vi "ecg_ncs_v1a.vi"() -> ()   [LabVIEW 2016]
uses:
  <instrlib>/niUSRP/niUSRP Timestamp.ctl
  C:/Program Files/National Instruments/LabVIEW 2016/examples/Instrument IO/Serial/support/Serial - Settings.ctl
  <vilib>/Analysis/coordinate.llb/Wrap Angle (array).vi
  <instrlib>/niUSRP/niUSRP Configure Time Start Trigger.vi
  <vilib>/Instr/_visa.llb/VISA Configure Serial Port (Instr).vi
  <instrlib>/niUSRP/niUSRP Fetch Rx Data (2D CDB).vi
  <vilib>/Analysis/3filter.llb/Butterworth Filter (DBL).vi
  <instrlib>/niUSRP/niUSRP Write Tx Data (2D CDB).vi
  <vilib>/measure/NI_MABase.lvlib
  <vilib>/Analysis/NI_AALBase.lvlib
  <vilib>/Analysis/NI_AALPro.lvlib
  <vilib>/Analysis/NI_AAL_Angle.lvlib
panel:
  out "Iteration visa":i32=2074
  in  "?":enum32{"ECG", "Heart Rate"}(tab)
  out "BMD101 Reading":i16[](graph)=[10]
  out "Heart Rate":u8[](graph)=[100]
  in  "Read Count":u32=24
  out "return count":u32=8
  out "Poor Sensor Quality: \nSensor off":bool=TRUE
  out "Poor Sensor Quality: \nSensor on":bool
  out "Heart Rate 2":u16[](array[numeric])=[100]
  out "Stop Loop":bool=TRUE
  in  "Read":bool=TRUE
  in  "Stop":bool
  in  "Serial Settings":T1={"baud rate"=57600, "data bits"=8, "parity"=enum."None", "stop bits"=10, "flow control"=0} {"flow control" items=["None"=0, "XON/XOFF"=1, "RTS/CTS"=2, "DTR/DSR"=4]; "stop bits" items=["1.0"=10, "1.5"=15, "2.0"=20]; "data bits" min=5 max=8 step=1; "baud rate" items=["75"=75, "110"=110, "134"=134, "150"=150, "300"=300, "600"=600, "1200"=1200, "1800"=1800, "2400"=2400, "4800"=4800, "7200"=7200, "9600"=9600, "14400"=14400, "19200"=19200, "28800"=28800, "38400"=38400, "56000"=56000, "57600"=57600, "115200"=115200, "128000"=128000, "230400"=230400]}
  in  "VISA resource name":refnum<visa-resource-name>="bmd101"
  in  "File Name":string="Test"
  in  "order1":i32=5
  in  "Path":path=path "D:/Research/SummerFall17Spring18/CnC/NCS/EcgNcsCorrelation"
  in  "Low-Pass Freq":dbl=200.0 format="%#_13g"
  in  "Sampling Rate":i32=500
  out "Gain":dbl=-15.0
  out "Bandwidth":dbl=56000000.0
  out "Coerced Carrier Frequency":dbl=2000000000.0 format="%#.17g"
  out "Coerced Tx IQ rate":dbl=1000000.0
  out "Coerced Rx IQ rate":dbl=1000000.0
  out "error IO":errorcluster={"status"=FALSE, "code"=-1074118647, "source"=""}
  in  "Rx Number of Samples":i32=20000
  in  "Tab Control 2":enum32{"NI-294x/295x", "NI-2900/2901"}(tab)=enum."NI-2900/2901"
  in  "channel 0 carrier\n frequency [Hz]":dbl=2000000000.0 format="%#_6p"
  in  "Rx carrier frequency [Hz]":dbl=2000000000.0 format="%#_6p"
  in  "Tx carrier frequency [Hz]":dbl=1000000000.0 format="%#_6p"
  in  "Start Trigger Time":T2={"whole seconds"=1, "fractional seconds"=0.0}
  out "Tx Active Antenna":string="TX1"
  in  "Tab Control":T3(tab)
  out "NCS tag Amp":dbl[](graph)=[0.013332788438327721, 0.0131552898712497, 0.012994905519721597, 0.012986271887777701, 0.013075284595455733, 0.013191204808537919, 0.013351894528100879, 0.01345386740636616, 0.013382234051438232, 0.013180163786137358]
  out "NCS tag Phase":dbl[](graph)=[114.08993023907641, 111.82225141412982, 110.02998222947944, 109.41153055749608, 110.12587965469353, 112.16042160734105, 113.81215100166591, 114.51260226782536, 113.6206368361215, 111.46787264294511]
  out "IQ":dbl[][](graph)
  out "Tag Amp":dbl[](graph)
  out "Tag Phase":dbl[](graph)
  out "Tx Waveform Graph":waveform(dbl)[](graph)=[{"t0"=timestamp(0 s since 1904-01-01), "dt"=1e-06, "Y"=array[2000 elements]}, {"t0"=timestamp(0 s since 1904-01-01), "dt"=1e-06, "Y"=array[2000 elements]}]
  in  "Channel 0\nTone Amplitude":dbl=0.707 step=0.05 format="%#.6g"
  in  "Channel 0 \nTone Frequency":dbl=5000.0 format="%#_6p"
  in  "Waveform Size":dbl=2000.0
  in  "Rx Active Antenna":string="RX2"
  in  "Device Name":refnum<k15>="MyB200"
  in  "Tx Gain":dbl=28.0 format="%#_6f"
  in  "Tx IQ Rate":dbl=1000000.0 format="%#_6p"
  in  "Rx Gain":dbl=32.0 format="%#_6f"
  in  "Rx IQ Rate":dbl=1000000.0 format="%#_6p"
  # "Rx Settings"
  # "Tx Settings"
  # "Note that on the NI-2900 and NI-2901, both Rx channels share an LO and both Tx channels share an LO. However, on the NI-294x/295x devices, Rx and Tx of channel 0 share an LO and Rx and Tx of channel 1 share an LO."
  # "This Tx graph should always have end and start tied up since this is being sent in a loop continuously. Otherwise phase jumps will be noticed."
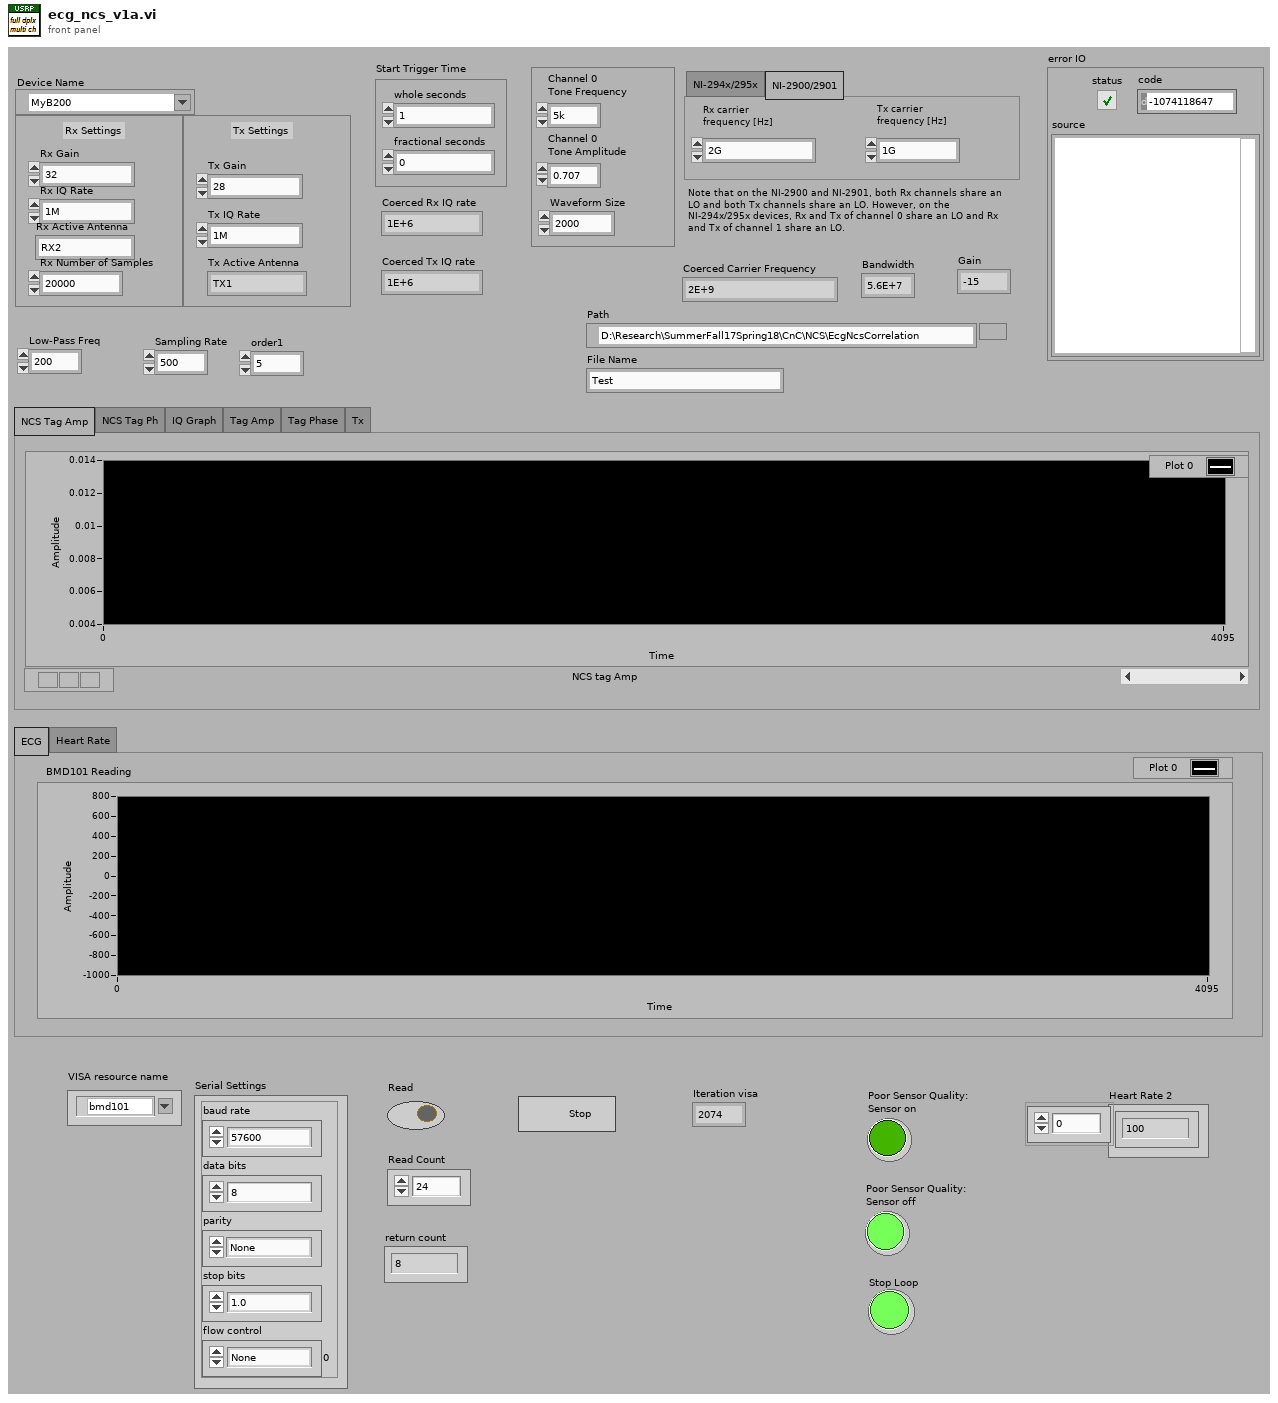
[diagram p1: front panel]
types:
  T1 = typedef "Serial - Settings.ctl" = cluster{"baud rate":u32, "data bits":u16, "parity":enum16{"None", "Odd", "Even", "Mark", "Space"}, "stop bits":u16, "flow control":u16}
  T2 = typedef "niUSRP Timestamp.ctl" = cluster{"whole seconds":u64, "fractional seconds":dbl}
  T3 = enum32{"NCS Tag Amp", "NCS Tag Ph", "IQ Graph", "Tag Amp", "Tag Phase", "Tx"}
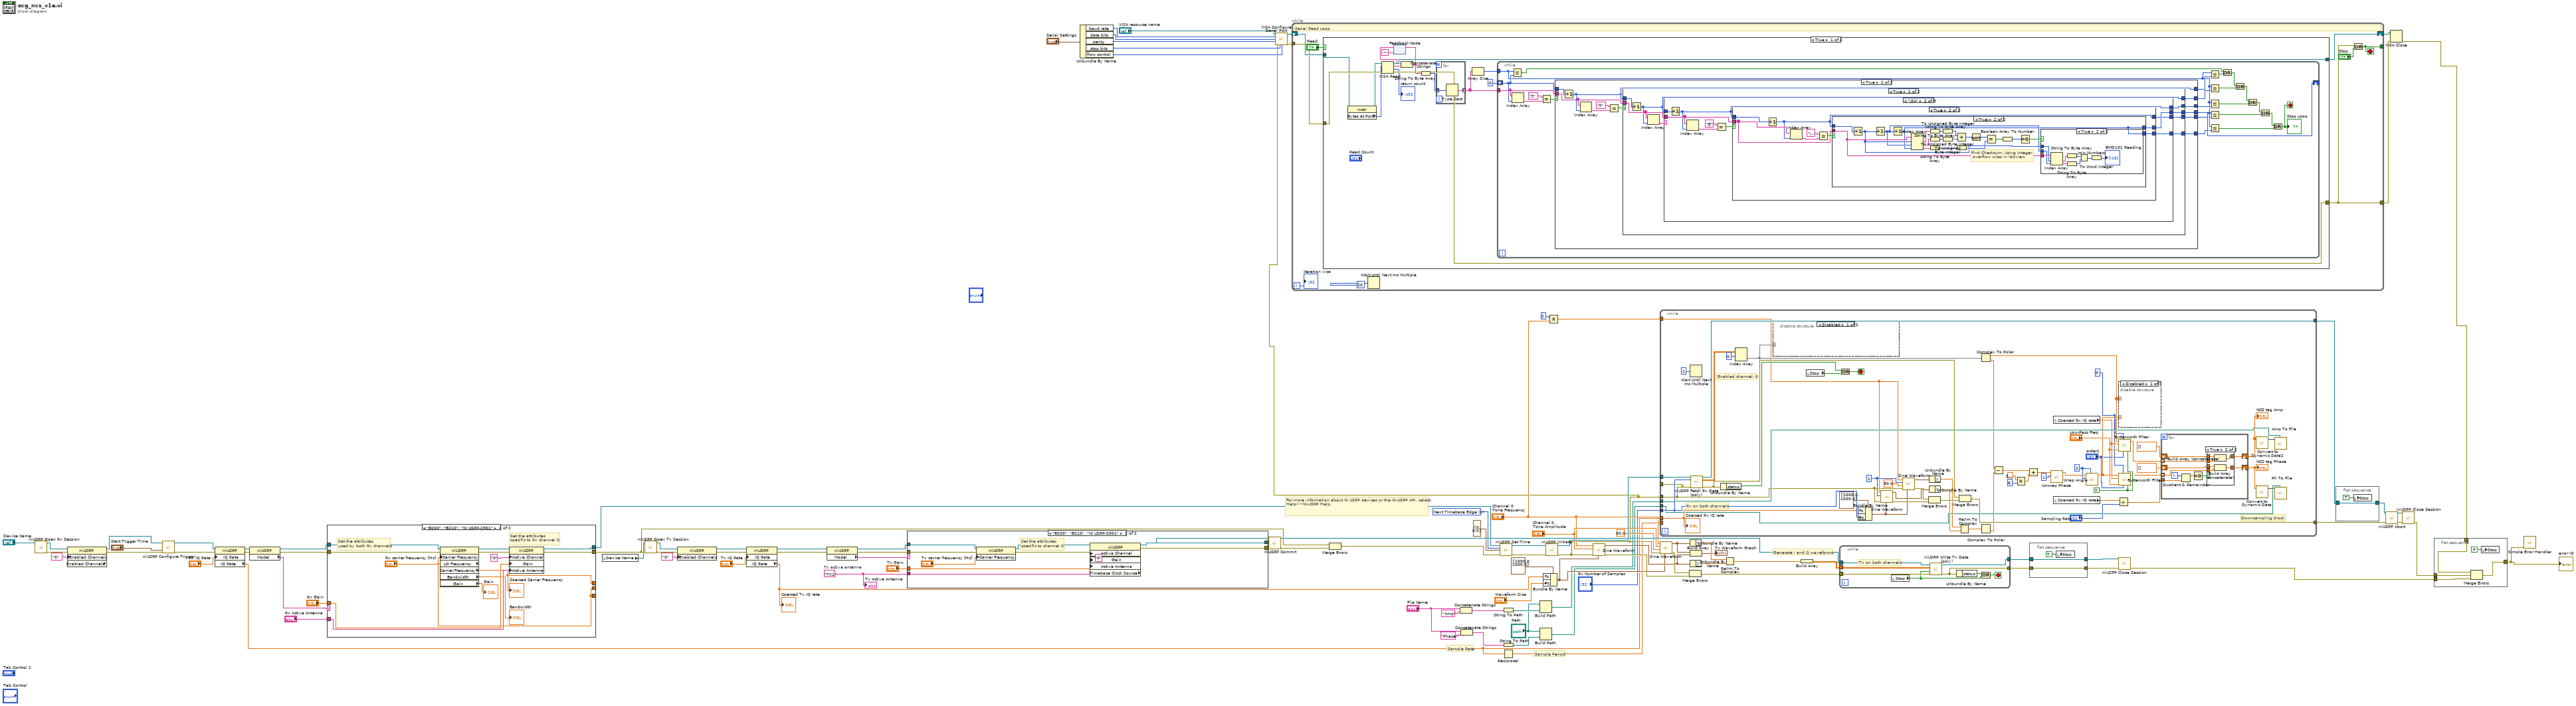
[diagram p0: block diagram]
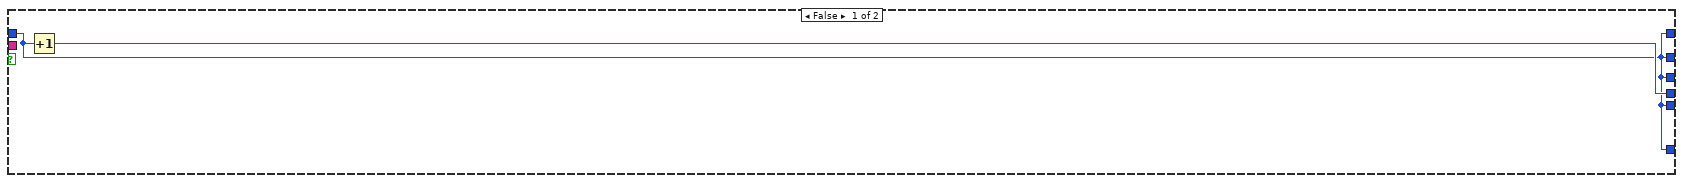
[diagram p2: hidden frame]
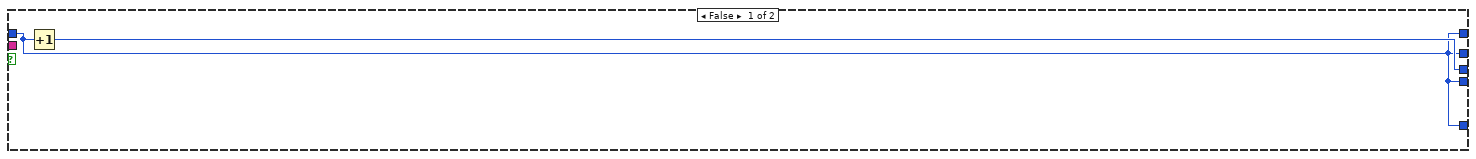
[diagram p3: hidden frame]
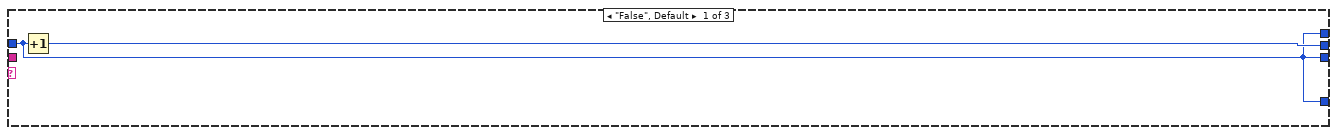
[diagram p4: hidden frame]
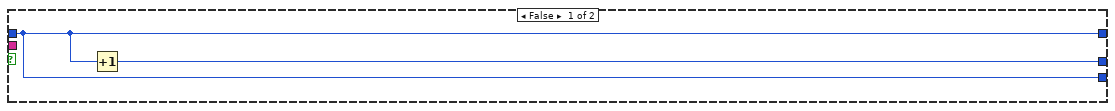
[diagram p5: hidden frame]
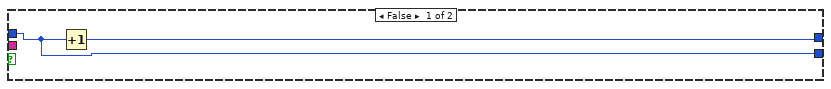
[diagram p6: hidden frame]
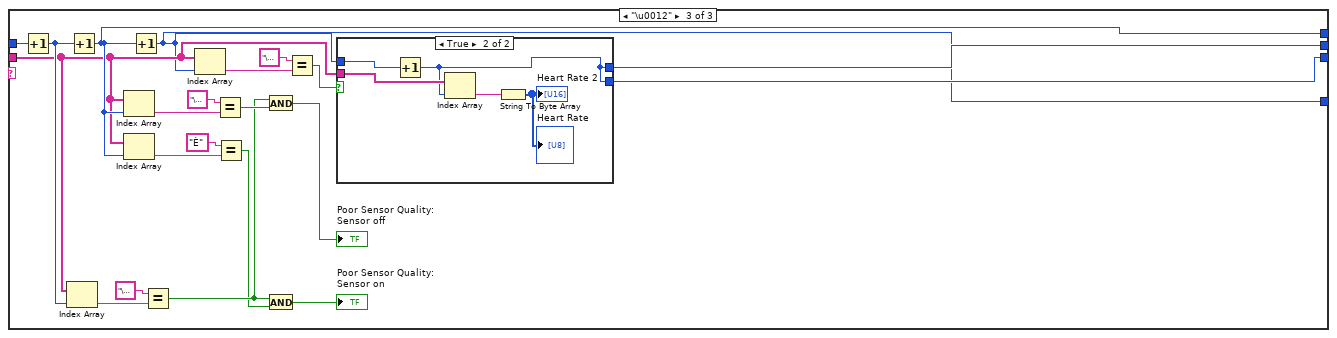
[diagram p8: hidden frame]
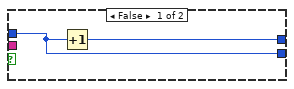
[diagram p9: hidden frame]
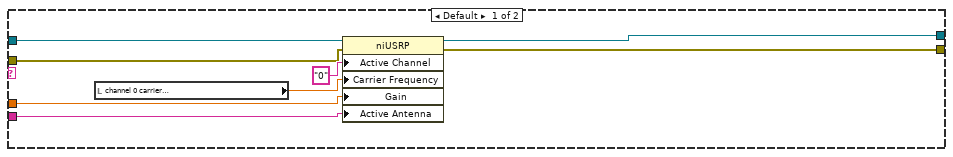
[diagram p11: hidden frame]
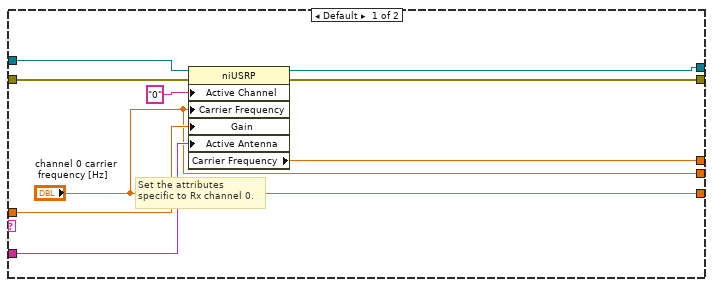
[diagram p12: hidden frame]
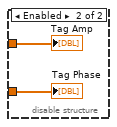
[diagram p13: hidden frame]
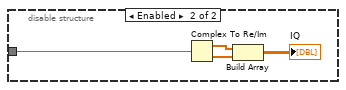
[diagram p14: hidden frame]
diagram:
  w73 = 1 items=["Now", "Next Timebase Edge"] ("apply timestamp")
  w42 = "TX1"  # Tx active antenna
  # "Sample Rate"
  # "Sample Period"
  # "For more information about NI USRP devices or the NI-USRP API, select Help>>NI-USRP Help."
  # "Generate I and Q waveforms."
  n1 = call <instrlib>:"niUSRP Open Rx Session.vi"("device names"="Device Name") -> ("session handle out"=w72:refnum<k15>, "error out"=w71:errorcluster)  [unwired: 13 in]
  n2 = property class="niUSRP" props=["Enabled Channels", "Enabled Channels"](reference=w72, error in=w71, "Enabled Channels"="0" ("Configuration:Enabled Channels")) -> (reference out=w70:refnum<k15>, error out=w69:errorcluster)  [unwired: 1 out]
  n3 = call-poly <instrlib>:"niUSRP Configure Trigger.vi"("session handle"=w70, "start trigger time"="Start Trigger Time", "error in (no error)"=w69) -> ("session handle out"=w66:refnum<k15>, "error out"=w65:errorcluster)  [unwired: 11 in]
  n4 = property class="niUSRP"(reference=w66, error in=w65, "IQ Rate"="Rx IQ Rate") -> (reference out=w62:refnum<k15>, error out=w63:errorcluster, "IQ Rate"=w29:dbl)
  n5 = property class="niUSRP"(reference=w62, error in=w63) -> (reference out=w57:refnum<k15>, error out=w58:errorcluster, "Model"=w59:string)
  n6 = case shown="\"B200\", \"B210\", \"NI USRP-2901\"" w59 {
    tunnel: w58 -> [w108 w118]
    tunnel: w57 -> [w107 w119]
    tunnel: [w104 w115] -> w61
    tunnel: [w103 w114] -> w60
    tunnel: "Rx Gain" -> [w106 w121]
    tunnel: "Rx Active Antenna" -> [w105 w120]
    tunnel: [w101 w110] -> _
    tunnel: ["channel 0 carrier\n frequency [Hz]" "Rx carrier frequency [Hz]"] -> _
    tunnel: ["channel 0 carrier\n frequency [Hz]" "Rx carrier frequency [Hz]"] -> _
    frame Default {
      # "Set the attributes \nspecific to Rx channel 0."
      n7 = property class="niUSRP"(reference=w107, error in=w108, "Active Channel"="0", "Carrier Frequency"="channel 0 carrier\n frequency [Hz]", "Gain"=w106, "Active Antenna"=w105) -> (reference out=w104:refnum<k15>, error out=w103:errorcluster, "Carrier Frequency"=w101:dbl)
    }
    frame "B200", "B210", "NI USRP-2901" {
      # "Set the attributes \nused by both Rx channels"
      # "Set the attributes \nspecific to Rx channel 0."
      n8 = property class="niUSRP" props=["Carrier Frequency", "LO Frequency", "Carrier Frequency", "Bandwidth", "Gain"](reference=w119, error in=w118, "Carrier Frequency"="Rx carrier frequency [Hz]") -> (reference out=w117:refnum<k15>, error out=w116:errorcluster, "Carrier Frequency"=w110:dbl, "Bandwidth"=→"Bandwidth":dbl, "Gain"=→"Gain":dbl)  [unwired: 1 out]
      "Coerced Carrier Frequency" <- w110
      n9 = property class="niUSRP"(reference=w117, error in=w116, "Active Channel"="0", "Gain"=w121, "Active Antenna"=w120) -> (reference out=w115:refnum<k15>, error out=w114:errorcluster)
    }
  }
  n10 = local read "Device Name"() -> (w94:refnum<k15>)
  n11 = call <instrlib>:"niUSRP Open Tx Session.vi"("device names"=w94, "error in (no error)"=w60) -> ("session handle out"=w68:refnum<k15>, "error out"=w67:errorcluster)  [unwired: 12 in]
  n12 = property class="niUSRP"(reference=w68, error in=w67, "Enabled Channels"="0" ("Configuration:Enabled Channels")) -> (reference out=w54:refnum<k15>, error out=w53:errorcluster)
  n13 = property class="niUSRP"(reference=w54, error in=w53, "IQ Rate"="Tx IQ Rate") -> (reference out=w48:refnum<k15>, error out=w49:errorcluster, "IQ Rate"=w46:dbl)
  "Coerced Tx IQ rate" <- w46
  n14 = property class="niUSRP"(reference=w48, error in=w49) -> (reference out=w50:refnum<k15>, error out=w51:errorcluster, "Model"=w47:string)
  n15 = case shown="\"B200\", \"B210\", \"NI USRP-2901\"" w47 {
    tunnel: "Tx Gain" -> [w130 w140]
    tunnel: w42 -> [w128 w138]
    tunnel: [w124 w132] -> w44
    tunnel: [w123 w131] -> w45
    tunnel: w51 -> [w127 w134]
    tunnel: w50 -> [w126 w137]
    frame Default {
      n16 = local read "channel 0 carrier\n frequency [Hz]"() -> (w125:dbl)
      n17 = property class="niUSRP"(reference=w126, error in=w127, "Active Channel"="0", "Carrier Frequency"=w125, "Gain"=w130, "Active Antenna"=w128) -> (reference out=w124:refnum<k15>, error out=w123:errorcluster)
    }
    frame "B200", "B210", "NI USRP-2901" {
      # "Set the attributes \nspecific to channel 0."
      n18 = property class="niUSRP"(reference=w137, error in=w134, "Carrier Frequency"="Tx carrier frequency [Hz]") -> (reference out=w136:refnum<k15>, error out=w135:errorcluster)
      n19 = property class="niUSRP" props=["Active Channel", "Gain", "Active Antenna", "Timebase Clock Source"](reference=w136, error in=w135, "Active Channel"="0", "Gain"=w140, "Active Antenna"=w138) -> (reference out=w132:refnum<k15>, error out=w131:errorcluster)  [unwired: 1 out]
    }
  }
  n20 = Unbundle By Name("Serial Settings") -> ("baud rate"=w13:u32, "data bits"=w12:u16, "parity"=w11:enum16{"None", "Odd", "Even", "Mark", "Space"}, "stop bits"=w10:u16, "flow control"=w9:u16)
  n21 = call <instrlib>:"niUSRP Commit.vi"("session handle"=w44, "error in (no error)"=w45) -> ("session handle out"=w96:refnum<k15>, "error out"=w97:errorcluster)  [unwired: 12 in]
  n22 = Merge Errors(w60, w97) -> (w75:errorcluster)
  n23 = Concatenate Strings("File Name", "Amp") -> (w22:string)
  n24 = Concatenate Strings("File Name", "Phase") -> (w18:string)
  n25 = call <instrlib>:"niUSRP Set Time.vi"("session handle"=w61, "apply timestamp"=w73, "timestamp"=T2 {"whole seconds"=0, "fractional seconds"=0.0}, "error in (no error)"=w75) -> ("session handle out"=w77:refnum<k15>, "error out"=w76:errorcluster)  [unwired: 10 in]
  n26 = String To Path(string=w22) -> (path=w21:path)
  n27 = String To Path(string=w18) -> (path=w17:path)
  n28 = Reciprocal(x=w29) -> (1/x=w80:dbl)
  n29 = Build Path(base path="Path", name or relative path=w21) -> (appended path=w24:path)
  n30 = Build Path(base path="Path", name or relative path=w17) -> (appended path=w15:path)
  n31 = Bundle By Name(cluster=cluster{"Fs":dbl, "#s":dbl} {"Fs"=1000.0, "#s"=1000.0} ("sampling info"), "Fs"=w46, "#s"="Waveform Size") -> (w79:cluster{"Fs":dbl, "#s":dbl})
  n32 = call <instrlib>:"niUSRP Initiate.vi"("session handle"=w77, "error in (no error)"=w76) -> ("session handle out"=w100:refnum<k15>, "error out"=w3:errorcluster)  [unwired: 12 in]
  n33 = call-poly "VISA Configure Serial Port"("VISA resource name"="VISA resource name", "baud rate (9600)"=w13, "data bits (8)"=w12, "parity (0:none)"=w11, "error in (no error)"=w3, "stop bits (10: 1 bit)"=w10, "flow control (0:none)"=w9) -> ("VISA resource name out"=w6:refnum<visa-resource-name>, "error out"=w5:errorcluster)  [unwired: 3 in, 4 out]
  n34 = while {
    shift-right: [w149] -> w7
    shift-left: w6 -> [w147]
    tunnel: w5 -> [w143]
    tunnel: [w146] -> _
    tunnel: [w142] -> w1
    i -> [w141]
    stop <- w146 stop-if-true
    # "Serial Read Loop"
    n35 = case shown="True" "Read" {
      tunnel: [w164 w293] -> w149
      tunnel: w147 -> [w152 w293]
      tunnel: [w153 w292] -> w142
      tunnel: w143 -> [w154 w292]
      frame True {
        n36 = property class="Instr"(reference=w152) -> (reference out=w151:refnum<visa-resource-name>, "Bytes at Port"=w150:u32)  [unwired: 1 in, 1 out]
        n37 = VISA Read(VISA resource name=w151, byte count=w150, error in (no error)=w154) -> (VISA resource name out=w164:refnum<visa-resource-name>, read buffer=w163:string, return count=→"return count":u32, error out=w153:errorcluster)
        n38 = feedback #1("") -> (w162:string)
        n39 = Concatenate Strings(w162, w163) -> (w159:string)
        n40 = feedback-in #1(w159) -> ()
        n41 = String To Byte Array(string=w159) -> (unsigned byte array=w160:u8[])
        n42 = for {
          tunnel: w160 -> [w291] mode=indexing
          tunnel: [w290] -> w157 mode=indexing
          n43 = Type Cast(x=w291) -> (*(type *) &x=w290:string)  [unwired: 1 in]
        }
        n44 = Array Size(array=w157) -> (size(s)=w155:i32)
        n45 = while {
          tunnel: w157 -> [w183]
          shift-right: [w187] -> _
          shift-left: 0 -> [w182]
          tunnel: w155 -> [w168]
          stop <- w165 stop-if-true
          n46 = Less Or Equal?(x=w168, y=w182) -> (x <= y?=w180:bool)
          n47 = Index Array(array=w183, index=w182) -> (element=w186:string)
          n48 = Equal?(x="ª", y=w186) -> (x = y?=w184:bool)
          n49 = case shown="True" w184 {
            tunnel: w182 -> [w188 w198]
            tunnel: [w189 w196] -> w187
            tunnel: w183 -> [_ w190]
            tunnel: [w188 w195] -> w181
            tunnel: [w188 w194] -> w178
            tunnel: [w188 w193] -> w175
            tunnel: [w188 w192] -> w172
            tunnel: [w188 w191] -> w169
            frame False {
              n50 = Increment(x=w188) -> (x+1=w189:i32)
            }
            frame True {
              n51 = Increment(x=w198) -> (x+1=w195:i32)
              n52 = Index Array(array=w190, index=w195) -> (element=w200:string)
              n53 = Equal?(x="ª", y=w200) -> (x = y?=w197:bool)
              n54 = case shown="True" w197 {
                tunnel: w195 -> [w201 w204]
                tunnel: [w202 w210] -> w196
                tunnel: w190 -> [_ w209]
                tunnel: [w201 w205] -> w194
                tunnel: [w201 w208] -> w193
                tunnel: [w201 w207] -> w192
                tunnel: [w201 w206] -> w191
                frame False {
                  n55 = Increment(x=w201) -> (x+1=w202:i32)
                }
                frame True {
                  n56 = Increment(x=w204) -> (x+1=w205:i32)
                  n57 = Index Array(array=w209, index=w205) -> (element=w203:string)
                  n58 = case shown="\"\\04\"" w203 {
                    tunnel: w205 -> [w211 w218 w281]
                    tunnel: [w212 w217 w263] -> w210
                    tunnel: w209 -> [_ w216 w265]
                    tunnel: [w211 w215 w267] -> w208
                    tunnel: [w211 w214 w264] -> w207
                    tunnel: [w211 w213 w262] -> w206
                    frame "False", Default {
                      n59 = Increment(x=w211) -> (x+1=w212:i32)
                    }
                    frame "\u0004" {
                      n60 = Increment(x=w218) -> (x+1=w215:i32)
                      n61 = Index Array(array=w216, index=w215) -> (element=w219:string)
                      n62 = Equal?(x="€", y=w219) -> (x = y?=w220:bool)
                      n63 = case shown="True" w220 {
                        tunnel: w215 -> [w222 w228]
                        tunnel: [w223 w227] -> w217
                        tunnel: w216 -> [_ w226]
                        tunnel: [w222 w225] -> w214
                        tunnel: [w222 w224] -> w213
                        frame False {
                          n64 = Increment(x=w222) -> (x+1=w223:i32)
                        }
                        frame True {
                          n65 = Increment(x=w228) -> (x+1=w225:i32)
                          n66 = Index Array(array=w226, index=w225) -> (element=w229:string)
                          n67 = Equal?(x="\u0002", y=w229) -> (x = y?=w230:bool)
                          n68 = case shown="True" w230 {
                            tunnel: w225 -> [w232 w237]
                            tunnel: [w233 w234] -> w227
                            tunnel: w226 -> [_ w238]
                            tunnel: [w232 w234] -> w224
                            frame False {
                              n69 = Increment(x=w232) -> (x+1=w233:i32)
                            }
                            frame True {
                              # "Find Checksum: Using Integer\n overflow rules in labview"
                              n70 = Increment(x=w237) -> (x+1=w236:i32)
                              n71 = Increment(x=w236) -> (x+1=w235:i32)
                              n72 = Increment(x=w235) -> (x+1=w234:i32)
                              n73 = Index Array(array=w238, index #1=w236, index #2=w235, index #3=w234) -> (element #1=w252:string, element #2=w251:string, element #3=w245:string)
                              n74 = String To Byte Array(string=w252) -> (unsigned byte array=w250:u8[])
                              n75 = String To Byte Array(string=w251) -> (unsigned byte array=w249:u8[])
                              n76 = String To Byte Array(string=w245) -> (unsigned byte array=w244:u8[])
                              n77 = To Unsigned Byte Integer(number=w250) -> (unsigned 8bit integer=w248:u8[])
                              n78 = To Unsigned Byte Integer(number=w249) -> (unsigned 8bit integer=w247:u8[])
                              n79 = Add(x=w248, y=w247) -> (x+y=w246:u8[])
                              n80 = To Unsigned Byte Integer(number=w244) -> (unsigned 8bit integer=w242:u8[])
                              n81 = Not(x=w246) -> (.not. x?=w243:u8[])
                              n82 = Equal?(x=w243, y=w242) -> (x = y?=w241:bool[])
                              n83 = Boolean Array To Number(Boolean array=w241) -> (number=w240:u32)
                              n84 = Equal To 0?(x=w240) -> (x = 0?=w239:bool)
                              n85 = case shown="True" w239 {
                                tunnel: w238 -> [_ w261]
                                tunnel: w236 -> [_ w254]
                                tunnel: w235 -> [_ w253]
                                frame False {
                                }
                                frame True {
                                n86 = Index Array(array=w261, index #1=w254, index #2=w253) -> (element #1=w260:string, element #2=w259:string)
                                n87 = String To Byte Array(string=w260) -> (unsigned byte array=w258:u8[])
                                n88 = String To Byte Array(string=w259) -> (unsigned byte array=w257:u8[])
                                n89 = Join Numbers(hi=w258, lo=w257) -> ((hi.lo)=w256:u16[])
                                n90 = To Word Integer(number=w256) -> (16bit integer=→"BMD101 Reading":i16[])
                                }
                              }
                            }
                          }
                        }
                      }
                    }
                    frame "\u0012" {
                      n91 = Increment(x=w281) -> (x+1=w277:i32)
                      n92 = Index Array(array=w265, index=w277) -> (element=w280:string)
                      n93 = Increment(x=w277) -> (x+1=w267:i32)
                      n94 = Index Array(array=w265, index=w267) -> (element=w278:string)
                      n95 = Index Array(array=w265, index=w267) -> (element=w275:string)
                      n96 = Increment(x=w267) -> (x+1=w262:i32)
                      n97 = Equal?(x="\u0002", y=w280) -> (x = y?=w272:bool)
                      n98 = Index Array(array=w265, index=w262) -> (element=w268:string)
                      n99 = Equal?(x="\u0000", y=w278) -> (x = y?=w274:bool)
                      n100 = Equal?(x="È", y=w275) -> (x = y?=w271:bool)
                      n101 = And(x=w272, y=w274) -> (x .and. y?=→"Poor Sensor Quality: \nSensor off":bool)
                      n102 = And(x=w272, y=w271) -> (x .and. y?=→"Poor Sensor Quality: \nSensor on":bool)
                      n103 = Equal?(x="\u0003", y=w268) -> (x = y?=w266:bool)
                      n104 = case shown="True" w266 {
                        tunnel: w262 -> [w283 w289]
                        tunnel: w265 -> [_ w288]
                        tunnel: [w283 w287] -> w264
                        tunnel: [w284 w287] -> w263
                        frame False {
                          n105 = Increment(x=w283) -> (x+1=w284:i32)
                        }
                        frame True {
                          n106 = Increment(x=w289) -> (x+1=w287:i32)
                          n107 = Index Array(array=w288, index=w287) -> (element=w286:string)
                          n108 = String To Byte Array(string=w286) -> (unsigned byte array=→"Heart Rate 2" →"Heart Rate":u8[])
                        }
                      }
                    }
                  }
                }
              }
            }
          }
          n109 = Less Or Equal?(x=w168, y=w181) -> (x <= y?=w179:bool)
          n110 = Less Or Equal?(x=w168, y=w178) -> (x <= y?=w176:bool)
          n111 = Less Or Equal?(x=w168, y=w175) -> (x <= y?=w173:bool)
          n112 = Less Or Equal?(x=w168, y=w172) -> (x <= y?=w170:bool)
          n113 = Less Or Equal?(x=w168, y=w169) -> (x <= y?=w166:bool)
          n114 = Or(x=w180, y=w179) -> (x .or. y?=w177:bool)
          n115 = Or(x=w177, y=w176) -> (x .or. y?=w174:bool)
          n116 = Or(x=w174, y=w173) -> (x .or. y?=w171:bool)
          n117 = Or(x=w171, y=w170) -> (x .or. y?=w167:bool)
          n118 = Or(x=w167, y=w166) -> (x .or. y?=w165:bool)
          "Stop Loop" <- w165
        }
      }
      frame False {
      }
    }
    n119 = Wait Until Next ms Multiple(millisecond multiple=u32 20 ("milliseconds to wait")) -> ()  [unwired: 1 out]
    n120 = Or(x=w142, y="Stop") -> (x .or. y?=w146:bool)
    "Iteration visa" <- w141
  }
  n121 = Multiply(x=2, y="Channel 0 \nTone Frequency") -> (x*y=w26:dbl)
  n122 = call <vilib>:"Sine Waveform.vi"("sampling info"=w79, "error in (no error)"=w3, "amplitude"="Channel 0\nTone Amplitude", "frequency"="Channel 0 \nTone Frequency") -> ("error out"=w41:errorcluster, "signal out"=w89:waveform(dbl))  [unwired: 6 in]
  n123 = while {
    tunnel: w100 -> [w350]
    tunnel: w3 -> [w295]
    tunnel: [w349] -> w35
    tunnel: w80 -> [_]
    tunnel: "Rx Number of Samples" -> [w345]
    tunnel: w29 -> [w336]
    tunnel: w26 -> [w337]
    tunnel: [w326] -> w25
    tunnel: w24 -> [w325]
    tunnel: w15 -> [w300]
    tunnel: [w295] -> _
    stop <- w327 stop-if-true
    w312 = 2 ("y")
    w305 = TRUE
    w307 = 0
    w343 = 1
    # "Downsampling block"
    # "Enabled channel: 0"
    # "Rx on both channels"
    n124 = Wait Until Next ms Multiple(millisecond multiple=u32 1 ("milliseconds to wait")) -> ()  [unwired: 1 out]
    n125 = call-poly <instrlib>:"niUSRP Fetch Rx Data (poly).vi"("session handle"=w350, "number of samples"=w345, "error in (no error)"=w295) -> ("session handle out"=w349:refnum<k15>, "data"=w334:cdb[][], "error out"=w331:errorcluster)  [unwired: 9 in, 1 out]
    n126 = Unbundle By Name(w331) -> ("status"=w348:bool)
    n127 = Index Array(array=w334, index (row)=0 ("y")) -> (element=w333:cdb[])  [unwired: 1 in]
    n128 = disable-structure shown="Disabled" {
      disable-tunnel: w333 -> [_ w353]
      frame Disabled {
      }
      frame Enabled {
        n129 = Complex To Re/Im(x + iy=w353) -> (x=w356:dbl[], y=w355:dbl[])
        n130 = Build Array(w356, w355) -> (→"IQ":dbl[][])
      }
    }
    n131 = local read "Stop"() -> (w294:bool)
    n132 = Or(x=w348, y=w294) -> (x .or. y?=w327:bool)
    n133 = Bundle By Name(cluster=cluster{"Fs":dbl, "#s":dbl} {"Fs"=1000.0, "#s"=1000.0} ("sampling info"), "Fs"=w336, "#s"=w345) -> (w342:cluster{"Fs":dbl, "#s":dbl})
    n134 = call <vilib>:"Sine Waveform.vi"("sampling info"=w342, "error in (no error)"=w295, "amplitude"=w343, "frequency"=w337) -> ("error out"=w341:errorcluster, "signal out"=w346:waveform(dbl))  [unwired: 6 in]
    n135 = call <vilib>:"Sine Waveform.vi"("sampling info"=w342, "error in (no error)"=w295, "phase"=90.0, "amplitude"=w343, "frequency"=w337) -> ("error out"=w340:errorcluster, "signal out"=w338:waveform(dbl))  [unwired: 5 in]
    n136 = Merge Errors(w340, w341) -> (w339:errorcluster)
    n137 = Unbundle By Name(w338) -> ("Y"=w322:dbl[])
    n138 = Unbundle By Name(w346) -> ("Y"=w321:dbl[])
    n139 = Re/Im To Complex(1:w321, 2:w322) -> (0:w315:cdb[])
    n140 = Merge Errors(w331, w339) -> (w326:errorcluster)
    n141 = Complex To Polar(r * e^(i*theta)=w333) -> (r=w324:dbl[], theta=w310:dbl[])
    n142 = Complex To Polar(r * e^(i*theta)=w315) -> (theta=w316:dbl[])  [unwired: 1 out]
    n143 = Subtract(x=w310, y=w316) -> (x-y=w314:dbl[])
    n144 = Multiply(x=3.141592653589793, y=6) -> (x*y=w317:dbl)
    n145 = Add(x=w314, y=w317) -> (x+y=w313:dbl[])
    n146 = call <vilib>:"Unwrap Phase.vi"("phase unit"=1 ("y"), "Phase"=w313) -> ("Unwrapped Phase"=w311:dbl[])  [unwired: 8 in, 1 out]
    n147 = local read "Coerced Rx IQ rate"() -> (w308:dbl)
    n148 = local read "Coerced Rx IQ rate"() -> (w330:dbl)
    n149 = call-poly <vilib>:"Wrap Angle.vi"("angle units"=w312, "angle range"=w312, "Angle In"=w311) -> ("Angle Out"=w309:dbl[])  [unwired: 7 in, 1 out]
    n150 = Divide(x=w330, y="Sampling Rate") -> (x/y=w328:dbl)
    n151 = disable-structure shown="Disabled" {
      disable-tunnel: w324 -> [_ w352]
      disable-tunnel: w309 -> [_ w351]
      frame Disabled {
      }
      frame Enabled {
        "Tag Amp" <- w352
        "Tag Phase" <- w351
      }
    }
    n152 = call-poly <vilib>:"Butterworth Filter.vi"("init/cont (init:F)"=w305, "order"="order1", "filter type"=w307, "low cutoff freq: fl"="Low-Pass Freq", "sampling freq: fs"=w308, "X"=w324) -> ("Filtered X"=w323:dbl[])  [unwired: 2 in, 1 out]
    n153 = call-poly <vilib>:"Butterworth Filter.vi"("init/cont (init:F)"=w305, "order"="order1", "filter type"=w307, "low cutoff freq: fl"="Low-Pass Freq", "sampling freq: fs"=w308, "X"=w309) -> ("Filtered X"=w303:dbl[])  [unwired: 2 in, 1 out]
    n154 = for {
      tunnel: w323 -> [w366] mode=indexing
      shift-right: [w364] -> w298
      shift-left: dbl[] [] -> [w365]
      tunnel: w328 -> [w360]
      shift-right: [w358] -> w301
      shift-left: dbl[] [] -> [w359]
      tunnel: w303 -> [w357] mode=indexing
      i -> [w363]
      n155 = Quotient & Remainder(x=w363, y=w360) -> (x-y*floor(x/y)=w361:dbl)  [unwired: 1 out]
      n156 = Equal To 0?(x=w361) -> (x = 0?=w362:bool)
      n157 = case shown="True" w362 {
        tunnel: w366 -> [_ w374]
        tunnel: w365 -> [w368 w373]
        tunnel: [w368 w372] -> w364
        tunnel: w359 -> [w367 w371]
        tunnel: [w367 w370] -> w358
        tunnel: w357 -> [_ w369]
        frame False {
        }
        frame True {
          n158 = Build Array (concatenate)(w373, w374) -> (w372:dbl[])
          n159 = Build Array (concatenate)(w371, w369) -> (w370:dbl[])
        }
      }
    }
    "NCS tag Amp" <- w298
    "NCS tag Phase" <- w301
    n160 = call "Convert to Dynamic Data2"("Array"=w298) -> ("Dynamic Data Type"=w297:dynamicdata)  [unwired: 3 in]
    n161 = call "Convert to Dynamic Data"("Array"=w301) -> ("Dynamic Data Type"=w302:dynamicdata)  [unwired: 3 in]
    n162 = call "Amp To File"("Signals"=w297, "Filename"=w325) -> ()  [unwired: 15 in, 3 out]
    n163 = call "Ph To File"("Signals"=w302, "Filename"=w300) -> ()  [unwired: 15 in, 3 out]
    "Coerced Rx IQ rate" <- w336
  }
  n164 = call <vilib>:"Sine Waveform.vi"("sampling info"=w79, "error in (no error)"=w3, "phase"=90.0, "amplitude"="Channel 0\nTone Amplitude", "frequency"="Channel 0 \nTone Frequency") -> ("error out"=w40:errorcluster, "signal out"=w88:waveform(dbl))  [unwired: 5 in]
  n165 = Merge Errors(w40, w41) -> (w39:errorcluster)
  n166 = Unbundle By Name(w88) -> ("Y"=w87:dbl[])
  n167 = Build Array(w88, w89) -> (→"Tx Waveform Graph":waveform(dbl)[])
  n168 = Unbundle By Name(w89) -> ("Y"=w86:dbl[])
  n169 = Re/Im To Complex(1:w86, 2:w87) -> (0:w82:cdb[])
  n170 = Build Array(w82) -> (w81:cdb[][])
  n171 = while {
    tunnel: w96 -> [w382]
    tunnel: w39 -> [w381]
    tunnel: [w379] -> w38
    tunnel: [w377] -> w33
    tunnel: w81 -> [w376]
    stop <- w378 stop-if-true
    # "Tx on both channels"
    n172 = local read "Stop"() -> (w375:bool)
    n173 = call-poly <instrlib>:"niUSRP Write Tx Data (poly).vi"("session handle"=w382, "data"=w376, "end of data?"=w375, "error in (no error)"=w381) -> ("session handle out"=w377:refnum<k15>, "error out"=w379:errorcluster)  [unwired: 10 in]
    n174 = Unbundle By Name(w379) -> ("status"=w380:bool)
    n175 = Compound Arithmetic op=OR(w380, w375) -> (w378:bool)
  }
  n176 = flat-sequence {
    tunnel: [w384] -> w37
    tunnel: w38 -> [w384]
    tunnel: [w383] -> w34
    tunnel: w33 -> [w383]
    frame #0 {
      n177 = local write "Stop"(TRUE ("STOP")) -> ()
    }
  }
  n178 = call <instrlib>:"niUSRP Close Session.vi"("session handle"=w34, "error in (no error)"=w37) -> ("error out"=w32:errorcluster)  [unwired: 13 in]
  n179 = flat-sequence {
    tunnel: [w386] -> w36
    tunnel: w35 -> [w386]
    frame #0 {
      n180 = local write "Stop"(TRUE ("STOP")) -> ()
    }
  }
  n181 = call <instrlib>:"niUSRP Abort.vi"("session handle"=w36, "error in (no error)"=w25) -> ("session handle out"=w93:refnum<k15>, "error out"=w92:errorcluster)  [unwired: 12 in]
  n182 = VISA Close(VISA resource name=w7, error in (no error)=w1) -> (error out=w4:errorcluster)
  n183 = call <instrlib>:"niUSRP Close Session.vi"("session handle"=w93, "error in (no error)"=w92) -> ("error out"=w30:errorcluster)  [unwired: 13 in]
  n184 = flat-sequence {
    tunnel: w32 -> [w391]
    tunnel: [w390] -> w2
    tunnel: w30 -> [w389]
    tunnel: w4 -> [w388]
    frame #0 {
      n185 = Merge Errors(w388, w389, w391) -> (w390:errorcluster)
      n186 = local write "Stop"(FALSE ("STOP")) -> ()
    }
  }
  n187 = call <vilib>:"Simple Error Handler.vi"("error in (no error)"=w2) -> ()  [unwired: 1 in, 8 out]
  "Tx Active Antenna" <- w42
  "error IO" <- w2
